vi "Configure Data Acquisition.vi"(0 "VISA resource name":refnum<visa-resource-name>, 1 "Stop Type (0: Count)":i32(ring) items=["Count", "Duration"], 2 "Sample Count (100 samples)":i32=100, 3 "Sample Duration (1 s)":i32=1, 5 "Function (0: DC Volts)":i32(ring) items=["DC Volts", "DC Current", "2-Wire Resistance", "4-Wire Resistance"], 7 "Manual Range (1.00)":dbl=1.0 format="%_3f", 9 "Sample Rate (9: 883/s)":i32(ring)=9 items=["1/10 m"=1, "1/5 m"=2, "1/m"=3, "1/10 s"=4, "1/s"=5, "10/s"=6, "50/s"=7, "100/s"=8, "833/s"=9, "1 k/s"=10, "5 k/s"=11, "10 k/s"=12, "50 k/s"=13], 11 "error in (no error)":errorcluster, 12 "Start Type (0: Auto)":i32(ring) items=["Auto", "External"], 13 "Delay Time (0 s)":i32) -> (4 "VISA resource name out":refnum<visa-resource-name>, 15 "error out":errorcluster)   [LabVIEW 2020, in "Library Instrument & Equipement.lvlib" / "Library Multimeter.lvlib" / "RIGOL DM3058.lvlib"]
doc: "Configure the data acquisition settings.\n\n<B>Note:</B>\nThis VI only applies for RIGOL DM3051 model with firmware 03.12.00.03.04.00.07 or later."
uses:
  RIGOL DM3058.lvlib
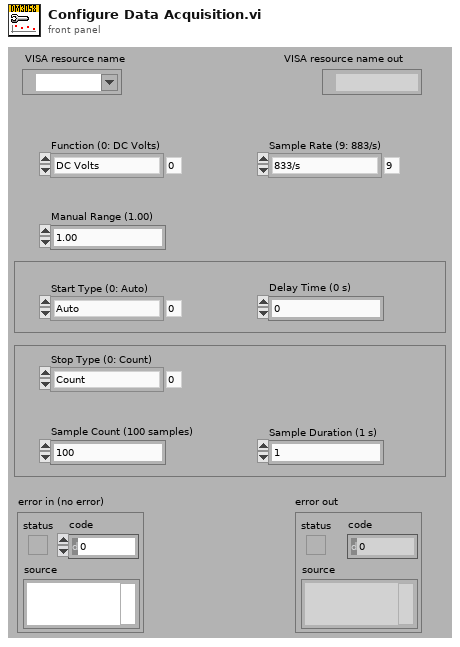
[diagram p1: front panel]
types:
  T1 = cluster{"DM Series Mode":u16, "Measurement Function":u16}
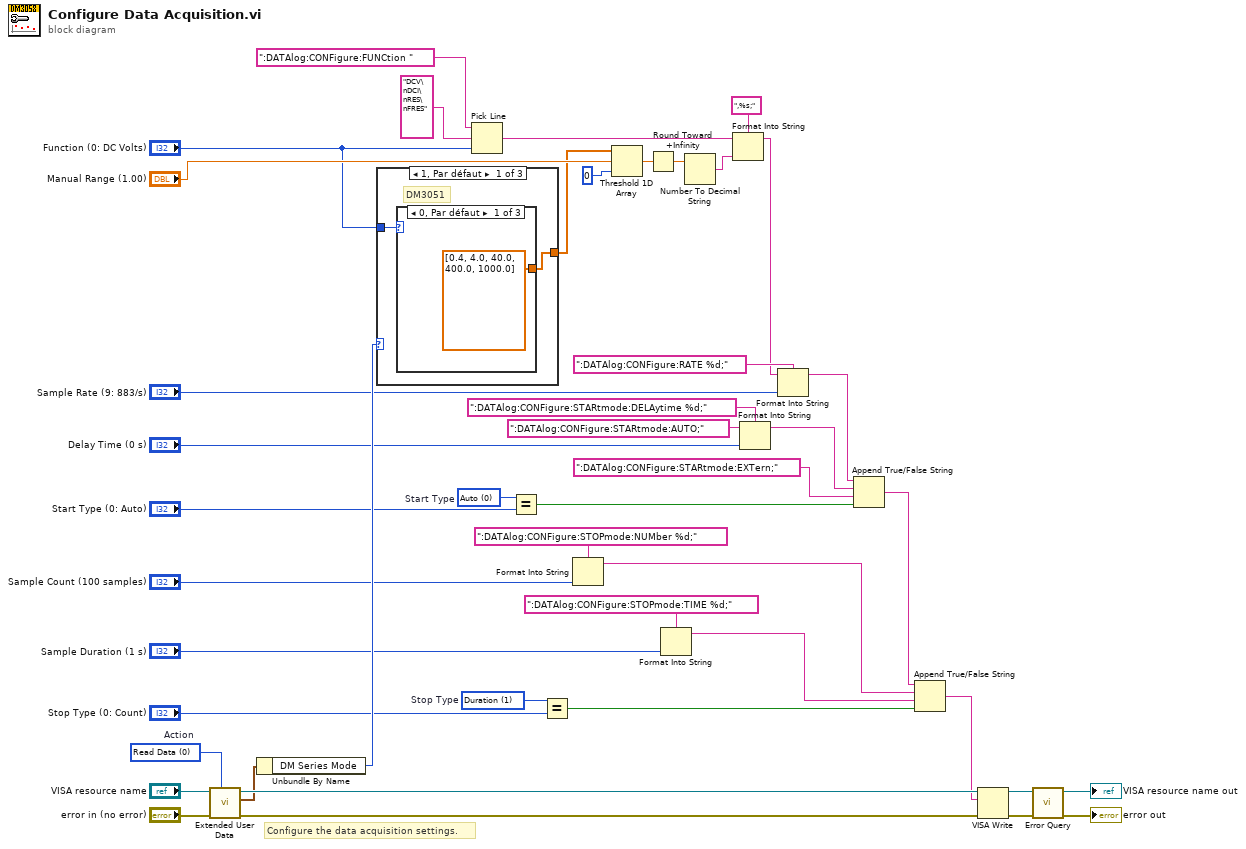
[diagram p0: block diagram]
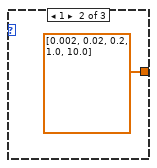
[diagram p2: hidden frame]
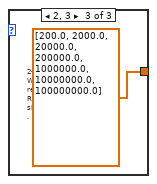
[diagram p3: hidden frame]
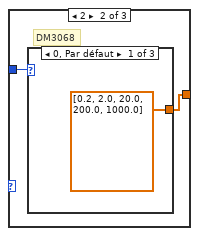
[diagram p4: hidden frame]
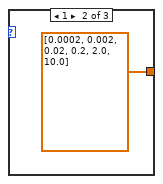
[diagram p5: hidden frame]
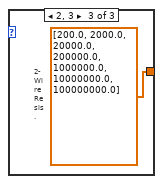
[diagram p6: hidden frame]
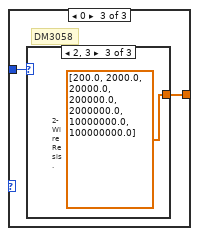
[diagram p7: hidden frame]
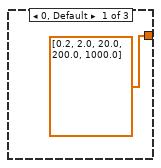
[diagram p8: hidden frame]
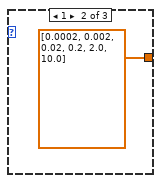
[diagram p9: hidden frame]
diagram:
  w16 = u16 1 items=["Count", "Duration"]  # Stop Type
  w21 = u16 0 items=["Auto", "External"]  # Start Type
  w37 = 0 items=["Read Data", "Write Data", "Clear Data", "Clear ALL Data"]  # Action
  # "Configure the data acquisition settings."
  n1 = call "Extended User Data.vi"("Action (1: Write Data)"=w37, "Error In (no error)"="error in (no error)", "VISA resource name in"="VISA resource name") -> ("Error Out"=w9:errorcluster, "User Data Out"=w1:T1, "VISA resource name out"=w10:refnum<visa-resource-name>)  [unwired: 1 in, 5 out]
  n2 = Unbundle By Name(w1) -> ("DM Series Mode"=w36:u16)
  n3 = case shown="1, Par défaut" w36 {
    tunnel: [w47 w51 w57] -> w34
    tunnel: "Function (0: DC Volts)" -> [w46 w52 w56]
    frame 1, Default {
      # "DM3051"
      n4 = case shown="0, Par défaut" w46 {
        tunnel: [dbl[] [0.4, 4.0, 40.0, 400.0, 1000.0] ("Array Constant") dbl[] [0.002, 0.02, 0.2, 1.0, 10.0] ("Array Constant") dbl[] [200.0, 2000.0, 20000.0, 200000.0, 1000000.0, 10000000.0, 100000000.0] ("Array Constant")] -> w47
        frame 0, Default {
          # "DC Voltage"
        }
        frame 1 {
          # "DC Current"
        }
        frame 2, 3 {
          # "4-Wire Resis."
          # "2-Wire Resis."
        }
      }
    }
    frame 2 {
      # "DM3068"
      n5 = case shown="0, Par défaut" w52 {
        tunnel: [dbl[] [0.2, 2.0, 20.0, 200.0, 1000.0] ("Array Constant") dbl[] [0.0002, 0.002, 0.02, 0.2, 2.0, 10.0] ("Array Constant") dbl[] [200.0, 2000.0, 20000.0, 200000.0, 1000000.0, 10000000.0, 100000000.0] ("Array Constant")] -> w51
        frame 0, Default {
          # "DC Voltage"
        }
        frame 1 {
          # "DC Current"
        }
        frame 2, 3 {
          # "4-Wire Resis."
          # "2-Wire Resis."
        }
      }
    }
    frame 0 {
      # "DM3058"
      n6 = case shown="2, 3" w56 {
        tunnel: [dbl[] [0.2, 2.0, 20.0, 200.0, 1000.0] ("Array Constant") dbl[] [0.0002, 0.002, 0.02, 0.2, 2.0, 10.0] ("Array Constant") dbl[] [200.0, 2000.0, 20000.0, 200000.0, 2000000.0, 10000000.0, 100000000.0] ("Array Constant")] -> w57
        frame 0, Default {
          # "DC Voltage"
        }
        frame 1 {
          # "DC Current"
        }
        frame 2, 3 {
          # "4-Wire Resis."
          # "2-Wire Resis."
        }
      }
    }
  }
  n7 = Pick Line(string ("")=":DATAlog:CONFigure:FUNCtion ", multi-line string="DCV\nDCI\nRES\nFRES", line index="Function (0: DC Volts)") -> (output string=w32:string)
  n8 = Equal?(x=w21, y="Start Type (0: Auto)") -> (x = y?=w19:bool)
  n9 = Equal?(x=w16, y="Stop Type (0: Count)") -> (x = y?=w14:bool)
  n10 = Format Into String(format string=":DATAlog:CONFigure:STOPmode:NUMber %d;", "Sample Count (100 samples)") -> (resulting string=w13:string)  [unwired: 2 in, 1 out]
  n11 = Threshold 1D Array(1:0 ("start index (0)"), 2:"Manual Range (1.00)", 3:w34) -> (0:w42:dbl)
  n12 = Round Toward +Infinity ("Round To +Infinity")(x=w42) -> (ceil(x): smallest int >= x=w41:dbl)
  n13 = Format Into String(format string=":DATAlog:CONFigure:STOPmode:TIME %d;", "Sample Duration (1 s)") -> (resulting string=w12:string)  [unwired: 2 in, 1 out]
  n14 = Number To Decimal String(number=w41) -> (decimal integer string=w31:string)  [unwired: 1 out]
  n15 = Format Into String(format string=",%s;", initial string=w32, w31) -> (resulting string=w28:string)  [unwired: 1 in, 1 out]
  n16 = Format Into String(format string=":DATAlog:CONFigure:STARtmode:DELAytime %d;", initial string=":DATAlog:CONFigure:STARtmode:AUTO;", "Delay Time (0 s)") -> (resulting string=w23:string)  [unwired: 1 in, 1 out]
  n17 = Format Into String(format string=":DATAlog:CONFigure:RATE %d;", initial string=w28, "Sample Rate (9: 883/s)") -> (resulting string=w22:string)  [unwired: 1 in, 1 out]
  n18 = Append True/False String(1:w19, 2:":DATAlog:CONFigure:STARtmode:EXTern;" ("false string"), 3:w23, 4:w22) -> (0:w11:string)
  n19 = Append True/False String(1:w14, 2:w12, 3:w13, 4:w11) -> (0:w4:string)
  n20 = VISA Write(VISA resource name=w10, write buffer=w4, error in (no error)=w9) -> (VISA resource name out=w8:refnum<visa-resource-name>, error out=w7:errorcluster)  [unwired: 1 out]
  n21 = call "Error Query.vi"("error in (no error)"=w7, "VISA resource name"=w8) -> ("error out"=→"error out":errorcluster, "VISA resource name out"=→"VISA resource name out":refnum<visa-resource-name>)  [unwired: 8 out]
